vi "JiLTest.vi"() -> ()   [LabVIEW 2010]
panel:
  out "time":dbl
  in  "doublein":dbl(slide) scale=-100.0..100.0
  out "doubleout":dbl
  in  "stringin":string="hola"
  in  "booleanin":bool
  out "booleanout":bool
  out "stringout":string="hola"
  in  "stop":bool
  out "intout":i32
  in  "intin":i32
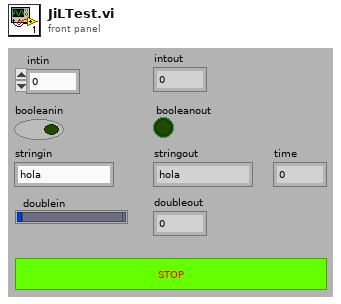
[diagram p1: front panel]
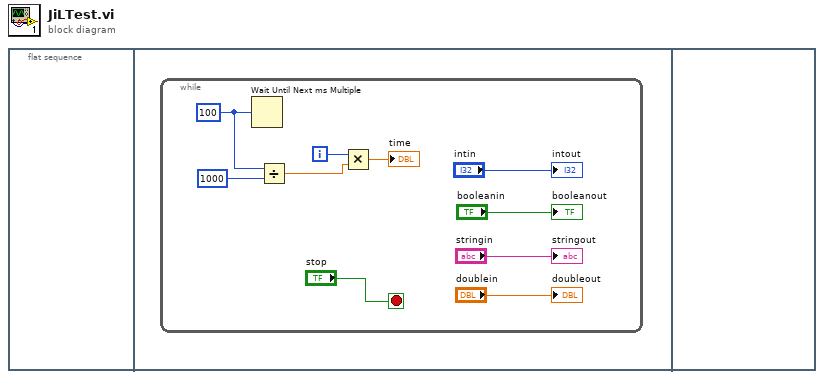
[diagram p0: block diagram]
diagram:
  n1 = flat-sequence {
    frame #0 {
    }
    frame #1 {
      n2 = while {
        i -> [w5]
        stop <- "stop" stop-if-true
        w6 = u32 100 ("millisecond multiple")
        n3 = Wait Until Next ms Multiple(millisecond multiple=w6) -> ()  [unwired: 1 out]
        n4 = Divide(x=w6, y=i64 1000) -> (x/y=w8:dbl)
        n5 = Multiply(x=w5, y=w8) -> (x*y=→"time":dbl)
        "intout" <- "intin"
        "stringout" <- "stringin"
        "booleanout" <- "booleanin"
        "doubleout" <- "doublein"
      }
    }
    frame #2 {
    }
  }
